vi "GT_BufDelay.vi"(8 "fifo":i16, 9 "delayTime":u16, 10 "Crd":i16, 11 "rtn_In":cluster{"rtn":i16, "Func":string}) -> (1 "fifo out":i16, 2 "Crd out":i16, 3 "rtn_Out":cluster{"rtn":i16, "Func":string})   [LabVIEW 2014]
uses:
  VC6/gts.dll
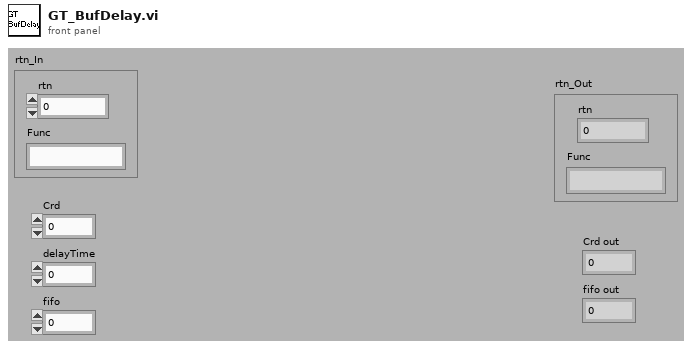
[diagram p1: front panel]
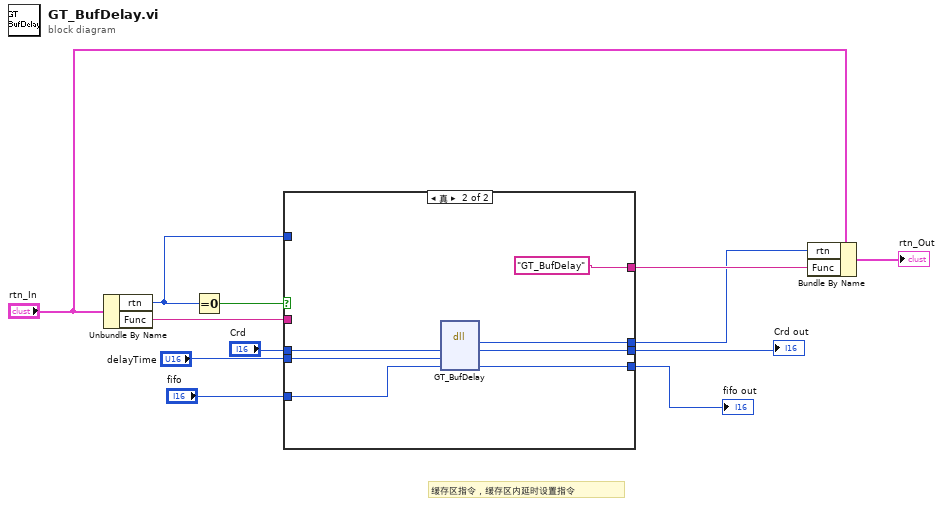
[diagram p0: block diagram]
diagram:
  # "缓存区指令，缓存区内延时设置指令"
  n1 = Unbundle By Name("rtn_In") -> ("rtn"=w7:i16, "Func"=w6:string)
  n2 = Equal To 0?(x=w7) -> (x = 0?=w12:bool)
  n3 = case shown="真" w12 {
    tunnel: [w15 "GT_BufDelay" ("Func")] -> w9
    tunnel: [w16 w22] -> w8
    tunnel: w7 -> [w16 _]
    tunnel: w6 -> [w15 _]
    tunnel: "Crd" -> [w14 w21]
    tunnel: "delayTime" -> [_ w20]
    tunnel: "fifo" -> [w13 w19]
    tunnel: [w14 w18] -> w2
    tunnel: [w13 w17] -> w1
    frame False {
    }
    frame True {
      n4 = dll-call lib="PTH2Fabs DNewGTS AC-800LWin7版源程序-20170926gts85VC6gts.dll" fn="GT_BufDelay"("Crd"=w21, "delayTime"=w20, "fifo"=w19) -> ("rtn"=w22:i16, "Crd"=w18:i16, "fifo"=w17:i16)  [unwired: 4 in, 2 out]
    }
  }
  "Crd out" <- w2
  "fifo out" <- w1
  n5 = Bundle By Name(cluster="rtn_In", "rtn"=w8, "Func"=w9) -> (→"rtn_Out":cluster{"rtn":i16, "Func":string})
